vi "Get DO Status - Multiple.vi"(0 "reference in":refnum<class "DO.lvclass">, 2 "DO Channel Numbers (Zero Based)":i32[](array[numeric]), 5 "error in (no error)":errorcluster) -> (14 "reference out":refnum<class "DO.lvclass">, 17 "DO Channel Status":bool[](array[boolean]), 19 "error out":errorcluster)   [LabVIEW 2017, in "DO.lvclass"]
uses:
  DO.lvclass
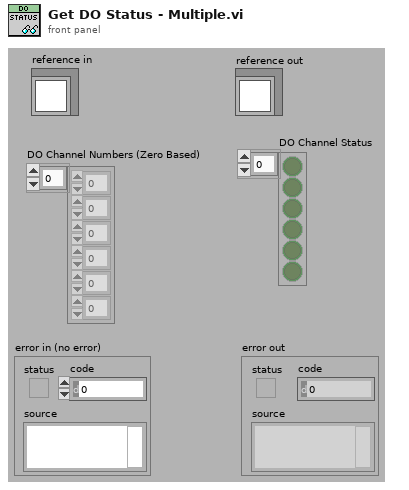
[diagram p1: front panel]
types:
  T1 = typedef "DO.lvclass/ObjectAttributes.ctl" = cluster{"DO Task":refnum<k21>, "DO Module Names (NI-Max Name)":string[], "Number of Channels Per DO Module":i32[], "DO Status":bool[], "Number of DO Modules":u32, "DO Status to Set":bool[], "DO On/Off Status":bool, "DO VI Reference":refnum<vi>, "Number of Total DO Channels":u32}
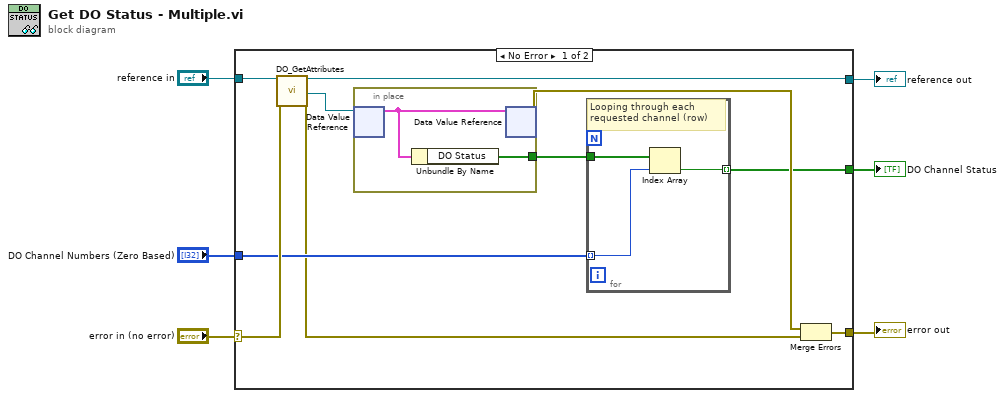
[diagram p0: block diagram]
diagram:
  n1 = case shown="No Error" "error in (no error)" {
    selector: "error in (no error)" -> [w15 w23]
    tunnel: [w12 w23] -> w5
    tunnel: [w13 w22] -> w3
    tunnel: "reference in" -> [w16 w22]
    tunnel: "DO Channel Numbers (Zero Based)" -> [w9 _]
    tunnel: [w8 _] -> w1
    frame No Error {
      n2 = call "DO_GetAttributes.vi"("reference in"=w16, "error in (no error)"=w15) -> ("reference out"=w13:refnum<class "DO.lvclass">, "DataRef"=w11:refnum<data-value>, "error out"=w7:errorcluster)  [unwired: 14 in, 1 out]
      n3 = in-place {
        in-place-border: [w17] -> w10
        n4 = in-place-dvr #1(w11) -> (w18:T1)  [unwired: 1 out]
        n5 = Unbundle By Name(w18) -> ("DO Status"=w17:bool[])
        n6 = in-place-dvr #1(w18) -> (w14:errorcluster)  [unwired: 1 out]
      }
      n7 = for {
        tunnel: w10 -> [w21]
        tunnel: w9 -> [w20] mode=indexing
        tunnel: [w19] -> w8 mode=indexing
        # "Looping through each requested channel (row)"
        n8 = Index Array(array=w21, index=w20) -> (element=w19:bool)
      }
      n9 = Merge Errors(w14, w7) -> (w12:errorcluster)
    }
    frame Error {
    }
  }
  "error out" <- w5
  "reference out" <- w3
  "DO Channel Status" <- w1
